vi "temp2.vi"() -> ()   [LabVIEW 2024]
uses:
  <vilib>/Instr/_visa.llb/VISA Configure Serial Port (Instr).vi
panel:
  in  "stop":bool
  out "read buffer":string
  in  "write buffer":string
  in  "VISA resource name":refnum<visa-resource-name>
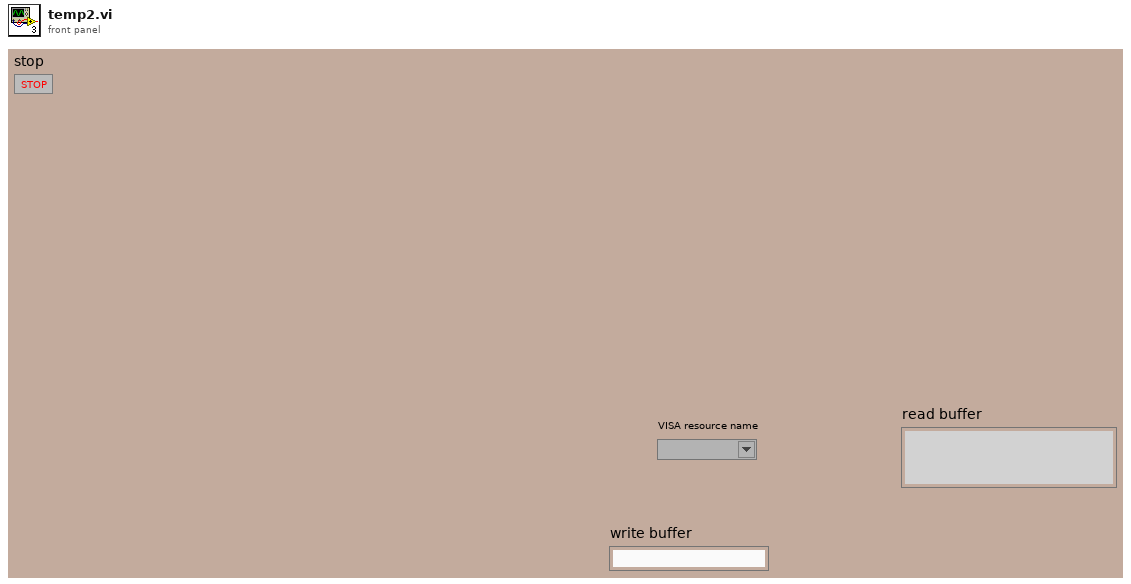
[diagram p1: front panel]
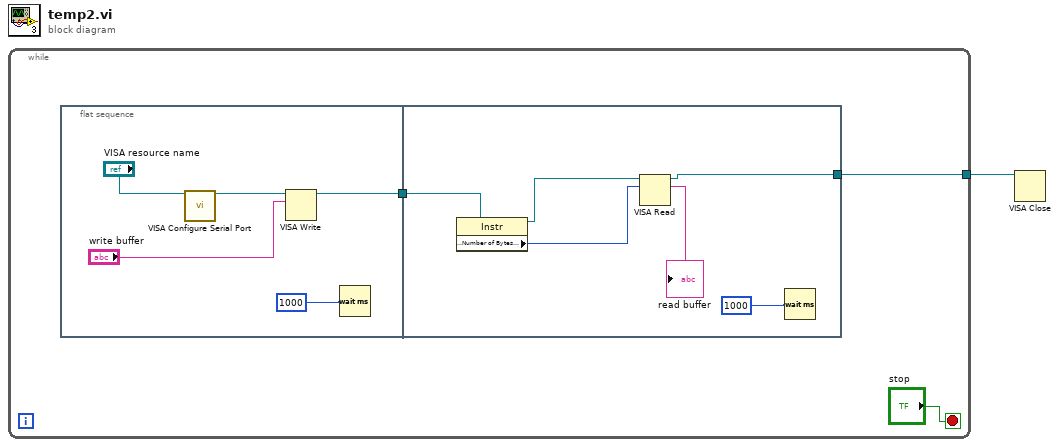
[diagram p0: block diagram]
diagram:
  n1 = while {
    tunnel: [w3] -> w1
    stop <- "stop" stop-if-true
    n2 = flat-sequence {
      tunnel: [w7] -> w4
      tunnel: w4 -> [w13]
      tunnel: [w11] -> w3
      frame #0 {
        n3 = call-poly "VISA Configure Serial Port"("VISA resource name"="VISA resource name") -> ("VISA resource name out"=w8:refnum<visa-resource-name>)  [unwired: 13 in, 1 out]
        n4 = VISA Write(VISA resource name=w8, write buffer="write buffer") -> (VISA resource name out=w7:refnum<visa-resource-name>)  [unwired: 1 in, 2 out]
        n5 = Wait (ms)(milliseconds to wait=u32 1000) -> ()  [unwired: 1 out]
      }
      frame #1 {
        n6 = property class="Instr"(reference=w13) -> (reference out=w15:refnum<visa-resource-name>, "Serial Settings:Number of Bytes at Serial Port"=w12:u32)  [unwired: 1 in, 1 out]
        n7 = VISA Read(VISA resource name=w15, byte count=w12) -> (VISA resource name out=w11:refnum<visa-resource-name>, read buffer=→"read buffer":string)  [unwired: 1 in, 2 out]
        n8 = Wait (ms)(milliseconds to wait=u32 1000) -> ()  [unwired: 1 out]
      }
    }
  }
  n9 = VISA Close(VISA resource name=w1) -> ()  [unwired: 1 in, 1 out]
